vi "Isc_libary.vi"(10 "Current":sgl[](array[numeric]), 11 "Voltage":sgl[](array[numeric])) -> (3 "Numeric":sgl)   [LabVIEW 2013]
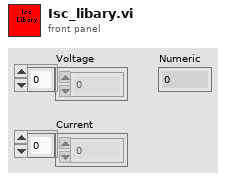
[diagram p1: front panel]
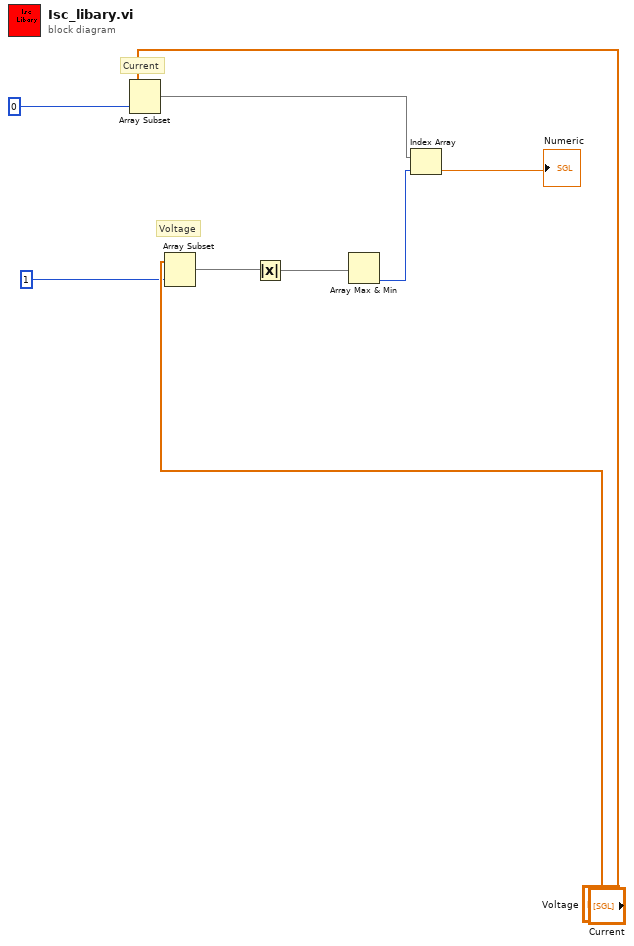
[diagram p0: block diagram]
diagram:
  # "Voltage"
  # "Current"
  n1 = Array Subset(array="Current", length=0 ("index")) -> (w3:sgl[])  [unwired: 1 in]
  n2 = Array Subset(array="Voltage", length=1 ("index")) -> (w5:sgl[])  [unwired: 1 in]
  n3 = Absolute Value(x=w5) -> (abs(x)=w4:sgl[])
  n4 = Array Max & Min(array=w4) -> (min index (indices)=w2:i32)  [unwired: 3 out]
  n5 = Index Array(array=w3, index=w2) -> (element=→"Numeric":sgl)
